vi "Build Context Menu.vi"(8 "error in (no error)":errorcluster, 10 "MenuRef":refnum<k9>, 11 "HIJ Vision Display in":refnum<class "HIJ Vision Display.lvclass">) -> (0 "error out":errorcluster, 2 "MenuRef out":refnum<k9>, 3 "HIJ Vision Display out":refnum<class "HIJ Vision Display.lvclass">)   [LabVIEW 2014, in "HIJ Vision Display.lvlib" / "HIJ Vision Display.lvclass"]
uses:
  HIJ Vision Display.lvclass
  HIJ Vision Display.lvclass/HIJ Vision Display.ctl
  Analyze/Results and Overlays/Results Base/Analyze Results Base.lvclass/Analyze Results Base.ctl
  Analyze/Results and Overlays/Results Base/Read Overlay_.vi
  Analyze/Results and Overlays/Results Base/Analyze Results Base.lvclass
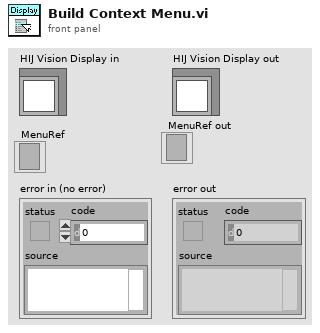
[diagram p1: front panel]
types:
  T1 = typedef "HIJ Vision Display.lvlib/HIJ Vision Display.lvclass/Named ROI.ctl" = cluster{"ROI":cluster{"Global Rectangle":i32[], "Contours":cluster{"Contour Type":u32, "ROI Type":u32, "Points":i32[]}[]}, "Name":string}
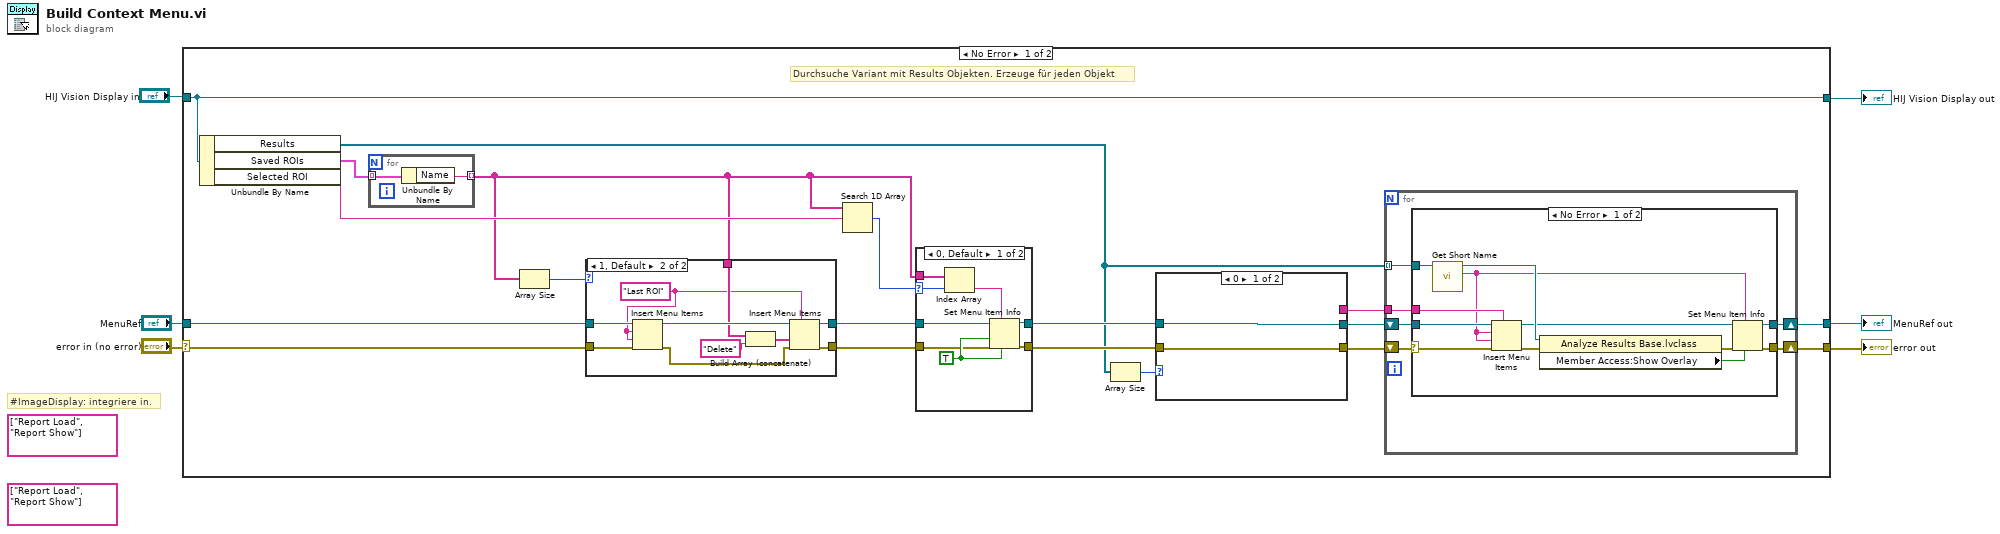
[diagram p0: block diagram]
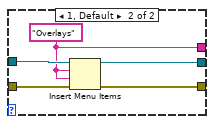
[diagram p2: hidden frame]
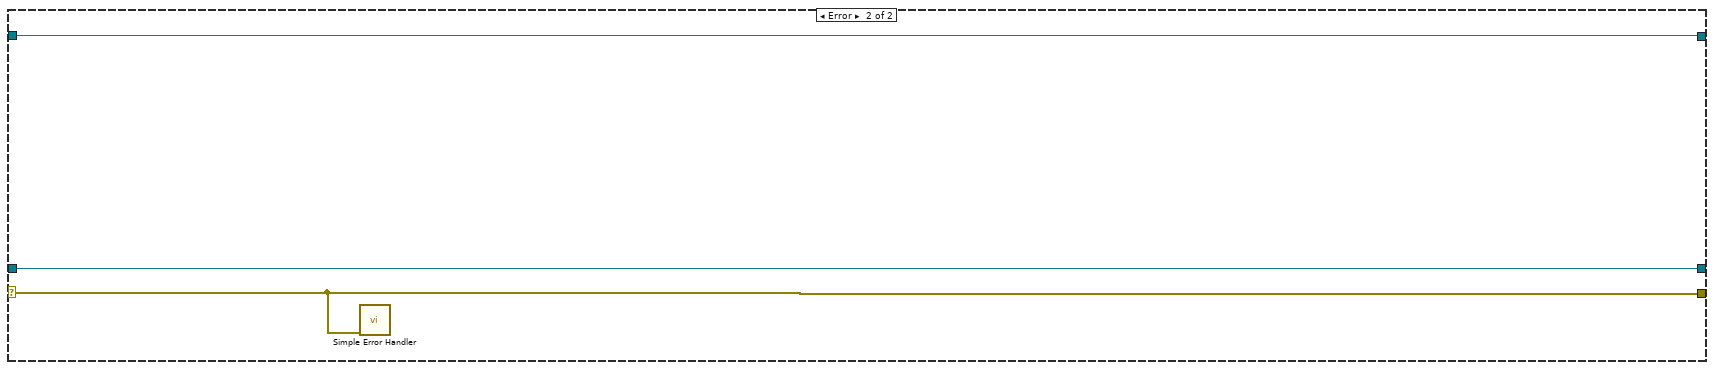
[diagram p6: hidden frame]
diagram:
  (unwired) string[] ["Report Load", "Report Show"] ("item names")
  (unwired) string[] ["Report Load", "Report Show"] ("item names")
  # "#ImageDisplay: integriere in."
  n1 = case shown="No Error" "error in (no error)" {
    selector: "error in (no error)" -> [w19 w77]
    tunnel: [w25 w79] -> w4
    tunnel: "HIJ Vision Display in" -> [w25 w79]
    tunnel: "MenuRef" -> [w16 w78]
    tunnel: [w12 w77] -> w2
    tunnel: [w13 w78] -> w1
    frame No Error {
      # "Durchsuche Variant mit Results Objekten. Erzeuge für jeden Objekt"
      n2 = Unbundle By Name(w25) -> ("Results"=w8:refnum<class "Analyze Results Base.lvclass">[], "Saved ROIs"=w24:T1[], "Selected ROI"=w23:string)
      n3 = for {
        tunnel: w24 -> [w76] mode=indexing
        tunnel: [w75] -> w22 mode=indexing
        n4 = Unbundle By Name(w76) -> ("Name"=w75:string)
      }
      n5 = Array Size(array=w22) -> (size(s)=w21:i32)
      n6 = case shown="1, Default" w21 {
        tunnel: w16 -> [w64 w73]
        tunnel: w22 -> [_ w70]
        tunnel: [w64 w69] -> w17
        tunnel: [w63 w68] -> w18
        tunnel: w19 -> [w63 w65]
        frame 0 {
        }
        frame 1, Default {
          w66 = "Last ROI" ("menu tag")
          n7 = Insert Menu Items(6:w65, 7:w66, 8:w66, 9:w73) -> (0:w74:errorcluster, 3:w72:refnum<k9>)  [unwired: 2 in, 1 out]
          n8 = Build Array (concatenate)(w70, "Delete" ("item names")) -> (w67:string[])
          n9 = Insert Menu Items(5:w66, 6:w74, 7:w67, 9:w72) -> (0:w68:errorcluster, 3:w69:refnum<k9>)  [unwired: 2 in, 1 out]
        }
      }
      n10 = Search 1D Array(1D array=w22, element=w23) -> (index of element=w20:i32)  [unwired: 1 in]
      n11 = case shown="0, Default" w20 {
        selector: w20 -> [w59 _]
        tunnel: w22 -> [w58 _]
        tunnel: w17 -> [w60 w61]
        tunnel: w18 -> [w55 w62]
        tunnel: [w54 w62] -> w10
        tunnel: [w53 w61] -> w11
        frame 0, Default {
          w56 = TRUE ("checked")
          n12 = Index Array(array=w58, index=w59) -> (element=w57:string)
          n13 = Set Menu Item Info(6:w56, 7:w57, 8:w55, 9:w56, 11:w60) -> (0:w54:errorcluster, 3:w53:refnum<k9>)  [unwired: 2 in]
        }
        frame -1 {
        }
      }
      n14 = Array Size(array=w8) -> (size(s)=w9:i32)
      n15 = case shown="0" w9 {
        tunnel: [w27 w29] -> w15
        tunnel: [w26 w30] -> w14
        tunnel: w11 -> [w26 w32]
        tunnel: w10 -> [w27 w31]
        tunnel: [_ w28] -> w7
        frame 0 {
        }
        frame 1, Default {
          w28 = "Overlays" ("menu tag")
          n16 = Insert Menu Items(6:w31, 7:w28, 8:w28, 9:w32) -> (0:w29:errorcluster, 3:w30:refnum<k9>)  [unwired: 2 in, 1 out]
        }
      }
      n17 = for {
        shift-right: [w36] -> w12
        shift-left: w15 -> [w34]
        shift-right: [w37] -> w13
        shift-left: w14 -> [w38]
        tunnel: w8 -> [w35] mode=indexing
        tunnel: w7 -> [w33]
        n18 = case shown="No Error" w34 {
          selector: w34 -> [w41 w52]
          tunnel: w35 -> [w46 _]
          tunnel: w38 -> [w44 w51]
          tunnel: [w50 w51] -> w37
          tunnel: [w47 w52] -> w36
          tunnel: w33 -> [w42 _]
          frame No Error {
            n19 = call-dynamic "Get Short Name.vi"("Analyze Results Base in"=w46) -> ("Short Name"=w39:string, "Analyze Results Base out"=w45:refnum<class "Analyze Results Base.lvclass">)  [unwired: 8 in, 1 out]
            n20 = Insert Menu Items(5:w42, 6:w41, 7:w39, 8:w39, 9:w44) -> (0:w40:errorcluster, 3:w43:refnum<k9>)  [unwired: 1 in, 1 out]
            n21 = property class="Analyze Results Base.lvclass"(reference=w45, error in=w40) -> (error out=w48:errorcluster, "Member Access:Show Overlay"=w49:bool)  [unwired: 1 out]
            n22 = Set Menu Item Info(6:w49, 7:w39, 8:w48, 11:w43) -> (0:w47:errorcluster, 3:w50:refnum<k9>)  [unwired: 3 in]
          }
          frame Error {
          }
        }
      }
    }
    frame Error {
      n23 = call <vilib>:"Simple Error Handler.vi"("error in (no error)"=w77) -> ()  [unwired: 4 in, 5 out]
    }
  }
  "error out" <- w2
  "HIJ Vision Display out" <- w4
  "MenuRef out" <- w1
